vi "1.vi"() -> ()   [LabVIEW 2026]
uses:
  <vilib>/express/express arith-compare/Formula/XNode/ExpressFormulaBlockNode.xnode
panel:
  out "Result 2":dbl
  out "Result":dbl
  out "output variable":dbl
  in  "Numeric 3":dbl
  in  "Numeric 2":dbl
  in  "Numeric":dbl
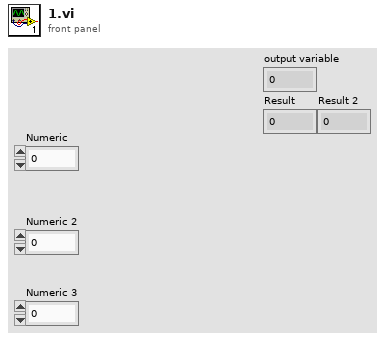
[diagram p1: front panel]
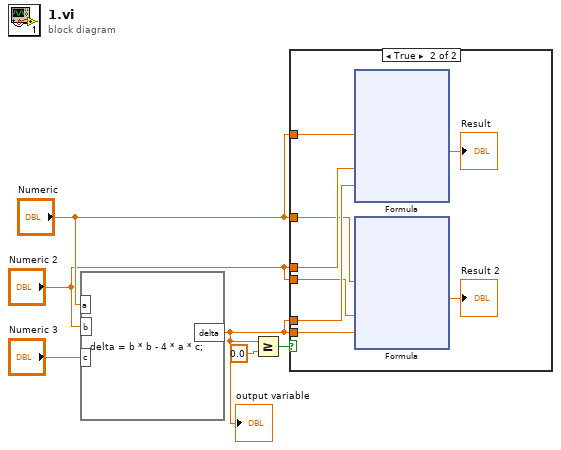
[diagram p0: block diagram]
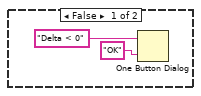
[diagram p2: hidden frame]
diagram:
  n1 = formula code="delta = b * b - 4 * a * c;"("a"="Numeric", "b"="Numeric 2", "c"="Numeric 3") -> ("delta"=w1:dbl)
  "output variable" <- w1
  n2 = Greater Or Equal?(x=w1, y=0.0) -> (x >= y?=w6:bool)
  n3 = case shown="True" w6 {
    tunnel: "Numeric" -> [_ w16]
    tunnel: "Numeric 2" -> [_ w15]
    tunnel: w1 -> [_ w14]
    tunnel: "Numeric" -> [_ w12]
    tunnel: "Numeric 2" -> [_ w11]
    tunnel: w1 -> [_ w10]
    frame False {
      n4 = One Button Dialog(message="Delta < 0", button name ("OK")="OK") -> ()  [unwired: 1 out]
    }
    frame True {
      n5 = xnode "Formula"("a"=w16, "b"=w15, "delta"=w14) -> ("Result"=→"Result":dbl)  [unwired: 1 in, 1 out]
      n6 = xnode "Formula"("a"=w12, "b"=w11, "delta"=w10) -> ("Result"=→"Result 2":dbl)  [unwired: 1 in, 1 out]
    }
  }
